vi "Wait DUT Load.vi"(8 "error in (no error)":errorcluster, 11 "Load?":bool) -> (0 "error out":errorcluster)   [LabVIEW 2024]
uses:
  Ctrl/PLC Enum.ctl
panel:
  out "Status?":bool
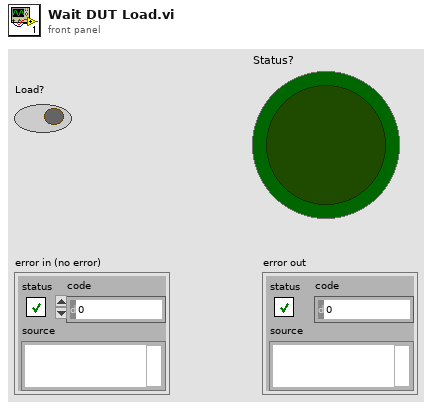
[diagram p1: front panel]
types:
  T1 = typedef "PLC Enum.ctl" = enum16{"Init", "Enable", "Orign", "Load", "Start", "Stop", "StartTest", "StopTest", "Reflector", "WriteResult", "SetSpeed", "SetOrign", "SetLoad", "ServoStatus?", "EquipStatus?", "Origin?", "TestStatus?", "Loadstatus?", "DUTStatus?", "Mes?", "Error？", "Position？", "Speed?", "PinCount", "RunMode", "SN", "Reset", "Jog+", "Jog-", "Close", "Up", "Down", "Clamp", "Release", "In", "Out", "EnterTestMode", "ExitTestMode", "StartButton", "ScanOK", "Power"}
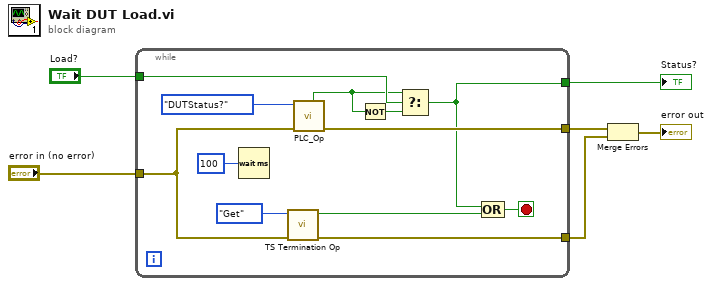
[diagram p0: block diagram]
diagram:
  n1 = while {
    tunnel: [w7] -> w6
    tunnel: "error in (no error)" -> [w13]
    tunnel: [w16] -> w5
    tunnel: [w12] -> w4
    tunnel: "Load?" -> [w10]
    stop <- w17 stop-if-true
    n2 = Wait (ms)(milliseconds to wait=u32 100 ("等待时间（毫秒）")) -> ()  [unwired: 1 out]
    n3 = call "TS Termination Op.vi"("error in (no error)"=w13, "Enum"=enum16{"Initialize", "Get", "Close"}."Get") -> ("error out"=w16:errorcluster, "Terminating or Aborting"=w15:bool)  [unwired: 8 in]
    n4 = call "PLC_Op.vi"("error in (no error)"=w13, "Status"=PLC_Enum."DUTStatus?") -> ("error out"=w12:errorcluster, "Boolean 2"=w9:bool)  [unwired: 4 in, 4 out]
    n5 = Not(x=w9) -> (.not. x?=w8:bool)
    n6 = Select(t=w9, s=w10, f=w8) -> (s? t:f=w7:bool)
    n7 = Compound Arithmetic op=OR(w7, w15) -> (w17:bool)
  }
  "Status?" <- w6
  n8 = Merge Errors(w4, w5) -> (→"error out":errorcluster)
